vi "Update.vi"(8 "error in (no error)":errorcluster, 11 "Object":refnum<class "Singleton.lvclass">) -> (0 "error out":errorcluster, 3 "Object (dup)":refnum<class "Singleton.lvclass">)   [LabVIEW 2014, in "Singleton.lvlib" / "Singleton.lvclass"]
uses:
  Singleton.lvclass
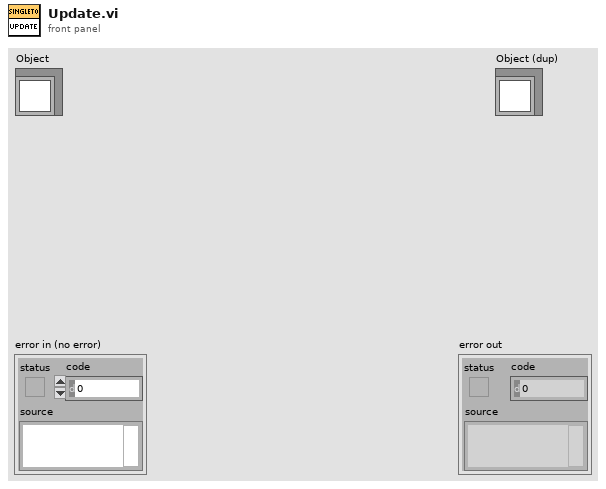
[diagram p1: front panel]
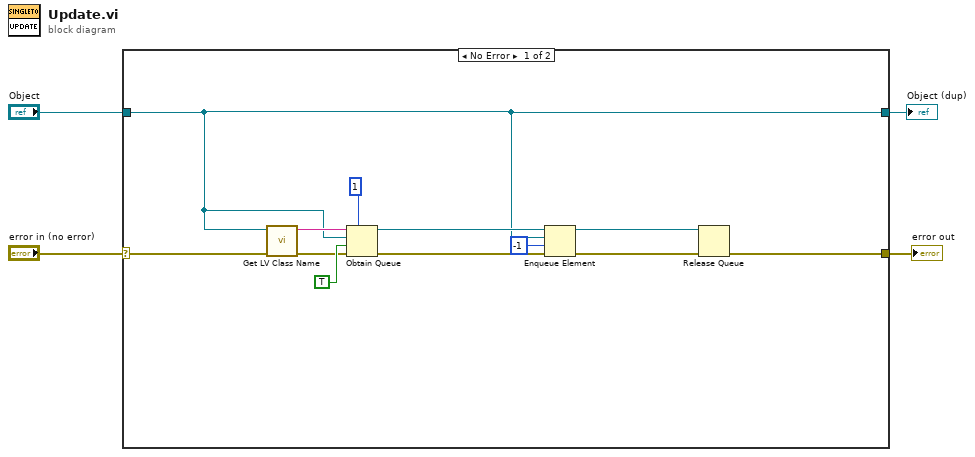
[diagram p0: block diagram]
diagram:
  n1 = case shown="No Error" "error in (no error)" {
    selector: "error in (no error)" -> [w13 w18]
    tunnel: [w6 w18] -> w3
    tunnel: "Object" -> [w9 w17]
    tunnel: [w9 w17] -> w1
    frame No Error {
      n2 = call <vilib>:"Get LV Class Name.vi"("error in (no error)"=w13, "object"=w9) -> ("error out"=w12:errorcluster, "class name"=w16:string)  [unwired: 8 in]
      n3 = Obtain Queue(max queue size (-1, unlimited)=1, name (unnamed)=w16, element data type=w9, create if not found? (T)=TRUE, error in (no error)=w12) -> (queue out=w11:refnum<queue>, error out=w10:errorcluster)  [unwired: 1 out]
      n4 = Enqueue Element(queue=w11, element=w9, timeout in ms (-1)=-1, error in (no error)=w10) -> (queue out=w7:refnum<queue>, error out=w8:errorcluster)  [unwired: 1 out]
      n5 = Release Queue(queue=w7, error in (no error)=w8) -> (error out=w6:errorcluster)  [unwired: 1 in, 2 out]
    }
    frame Error {
    }
  }
  "error out" <- w3
  "Object (dup)" <- w1
